vi "syrup-temp-tuner.vi"() -> ()   [LabVIEW 2013]
uses:
  <vilib>/Analysis/polynomials.llb/Scalar Polynomial Evaluation (DBL).vi
  <vilib>/Analysis/NI_AALPro.lvlib
panel:
  in  "Parameter Request":bool
  in  "Maximum Error (degF)":dbl=32.0 min=0.0 max=56.0 step=0.1
  in  "Temp Sim (degF)":dbl=32.0 min=32.0 max=1832.0 step=0.1 format="%.1f"
  in  "Hysteresis (degF)":dbl=32.0 min=0.0 max=56.0 step=0.1 format="%#.1f"
  in  "Valve Time Gain":u16=100
  in  "Min Valve On Time (ms)":u16=100
  in  "Open Valve":u8
  in  "Close Valve":u8
  in  "Auto Mode":bool
  in  "Valve On Time (ms)":u16=100
  in  "Write Tuning":bool
  in  "Temp Setpoint (degF)":dbl=32.0 min=32.0 max=1832.0 step=1.0
  out "Array":dbl[](array[numeric]) format="%.1f"
  in  "Write Setpoint":bool
  out "Waveform Chart":T1(graph)={"[0]"=63.3344, "[1]"=32.0, "[2]"=32.0, "[3]"=32.0, "[4]"=0.0, "[5]"=0.0, "[6]"=0.0, "[7]"=0.0, "[8]"=0.0}
  in  "stop":bool
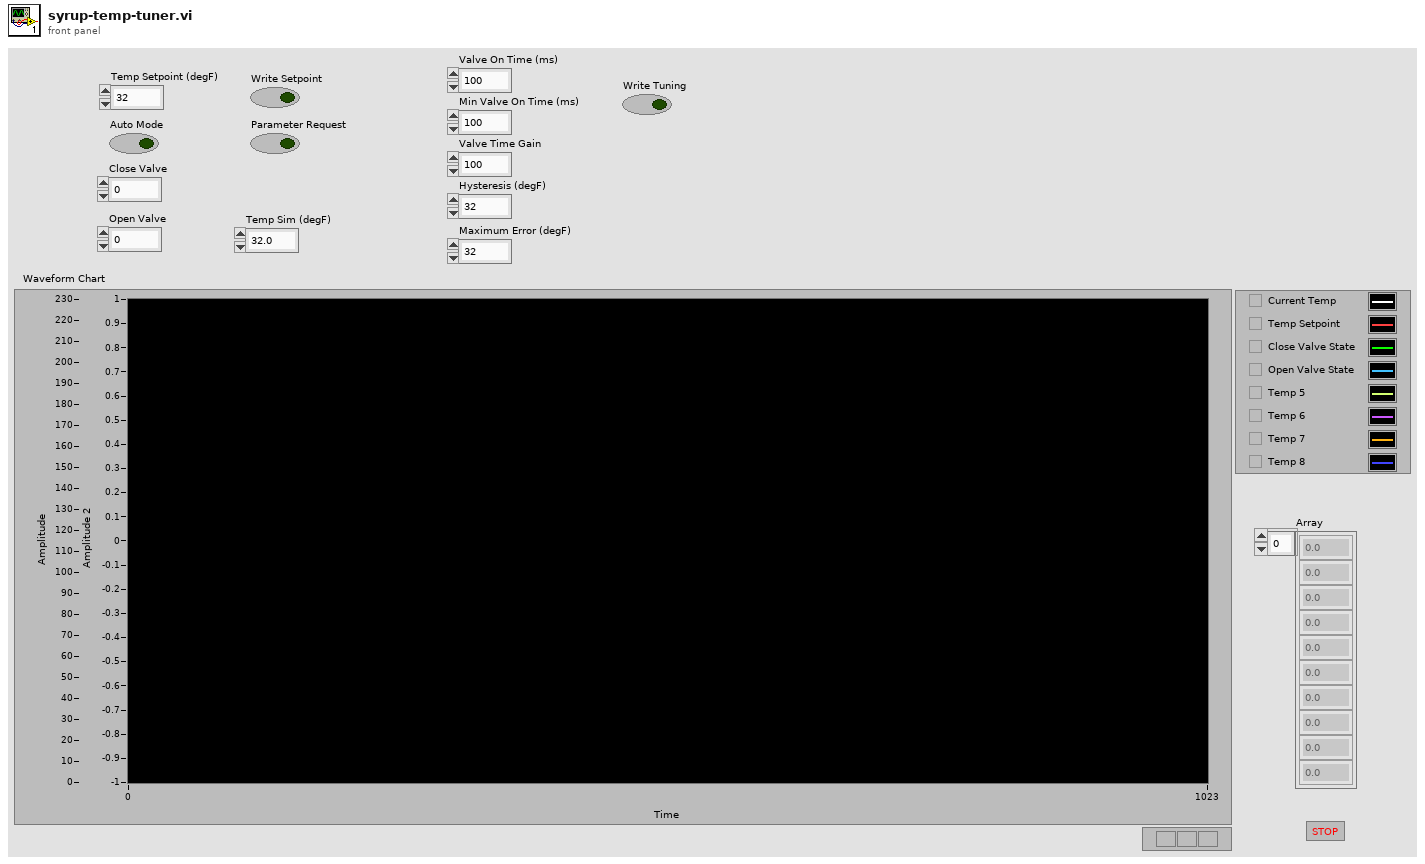
[diagram p1: front panel]
types:
  T1 = cluster{"[0]":dbl, "[1]":dbl, "[2]":dbl, "[3]":dbl, "[4]":dbl, "[5]":dbl, "[6]":dbl, "[7]":dbl, "[8]":dbl}
  T2 = enum16{"HSCAN", "MSCAN", "SWCAN", "LSFTCAN", "HSCAN2", "HSCAN3"}
  T3 = cluster{"DeviceType":i32, "Handle":i32, "NumberOfClients":i32, "SerialNumber":i32, "MaxAllowedClients":i32}[]
  T4 = cluster{"DeviceType":i32, "Handle":i32, "NumberOfClients":i32, "SerialNumber":i32, "MaxAllowedClients":i32}
  T5 = enum16{"DEVICE", "HSCAN", "MSCAN", "SWCAN", "LSFTCAN", "FORDSCP", "J1708", "JVPW", "ISO", "FIRE_HSCAN2", "FIRE_MSCAN1", "FIRE_HSCAN3", "FIRE_LIN2", "FIRE_LIN3", "FIRE_LIN4"}
  T6 = typedef "ctl spymessage.ctl" = cluster{"StatusBitField":u32, "StatusBitField2":u32, "TimeHardware":u32, "TimeHardware2":u32, "TimeSystem":u32, "TimeSystem2":u32, "TimeStampHardwareID":u8, "TimeStampHardwareID2":u8, "NetworkID":u8, "NodeID":u8, "Protocol":u8, "MessagePieceID":u8, "ColorID":u8, "NumberBytesHeader":u8, "NumberBytesData":u8, "DescriptionID":u16, "ArbIDOrHeader":u32, "Data [8]":u8[], "AckBytes [8]":u8[], "Value":sgl, "MiscData":u8}
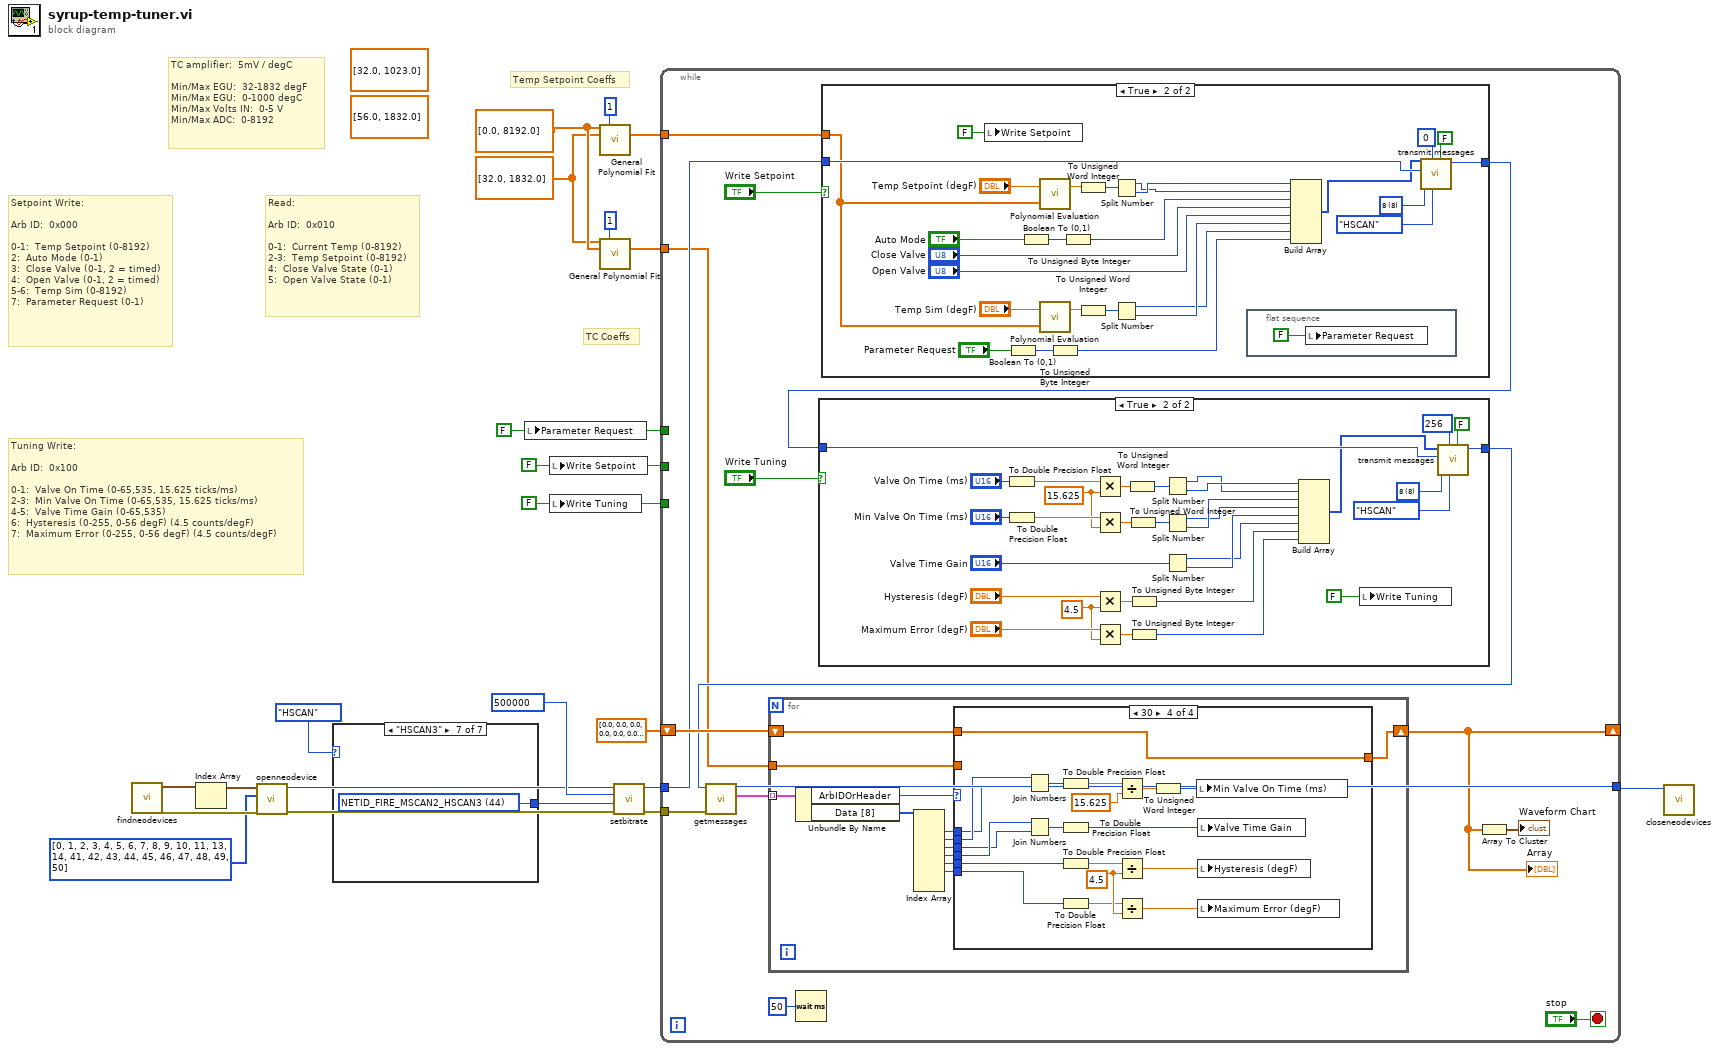
[diagram p0: block diagram]
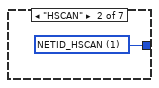
[diagram p3: hidden frame]
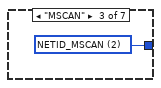
[diagram p4: hidden frame]
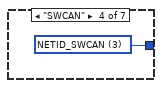
[diagram p5: hidden frame]
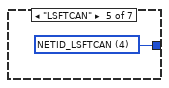
[diagram p6: hidden frame]
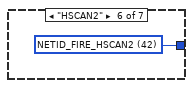
[diagram p7: hidden frame]
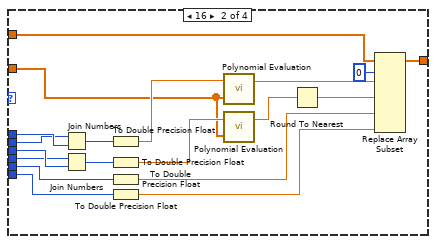
[diagram p11: hidden frame]
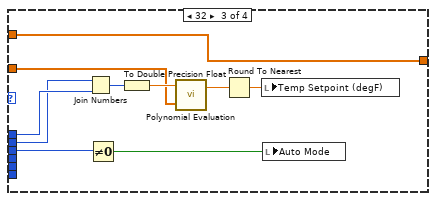
[diagram p12: hidden frame]
diagram:
  w1 = FALSE ("Send")
  (unwired) dbl[] [56.0, 1832.0] ("Y")
  (unwired) dbl[] [32.0, 1023.0] ("Y")
  w6 = FALSE ("Send")
  w2 = dbl[] [32.0, 1832.0] ("Y")
  w3 = dbl[] [0.0, 8192.0] ("Y")
  w9 = FALSE ("Send")
  w16 = 500000 items=["20000"=20000, "33333"=33333, "50000"=50000, "62500"=62500, "83333"=83333, "100000"=100000, "125000"=125000, "250000"=250000, "500000"=500000, "800000"=800000, "1000000"=1000000] ("Bit Rate")
  w19 = i8[] [0, 1, 2, 3, 4, 5, 6, 7, 8, 9, 10, 11, 13, 14, 41, 42, 43, 44, 45, 46, 47, 48, 49, 50] items=["NETID_DEVICE"=0, "NETID_HSCAN"=1, "NETID_MSCAN"=2, "NETID_SWCAN"=3, "NETID_LSFTCAN"=4, "NETID_FORDSCP"=5, "NETID_J1708"=6, "NETID_AUX"=7, "NETID_JVPW"=8, "NETID_ISO_LIN"=9, "NETID_ISOPIC"=10, "NETID_MAIN51"=11, "NETID_SCI"=13, "NETID_ISO2"=14, "NETID_FIRE_HSCAN1"=41, "NETID_FIRE_HSCAN2"=42, "NETID_FIRE_MSCAN1"=43, "NETID_FIRE_MSCAN2_HSCAN3"=44, "NETID_FIRE_SWCAN"=45, "NETID_FIRE_LSFT"=46, "NETID_FIRE_LIN1"=47, "NETID_FIRE_LIN2"=48, "NETID_FIRE_LIN3"=49, "NETID_FIRE_LIN4"=50] ("bNetworkIDs")
  # "Temp Setpoint Coeffs"
  # "TC Coeffs"
  # "TC amplifier:  5mV / degC\n\nMin/Max EGU:  32-1832 degF\nMin/Max EGU:  0-1000 degC\nMin/Max Volts IN:  0-5 V\nMin/Max ADC:  0-8192"
  # "Read:\n\nArb ID:  0x010\n\n0-1:  Current Temp (0-8192)\n2-3:  Temp Setpoint (0-8192)\n4:  Close Valve State (0-1)\n5:  Open Valve State (0-1)"
  # "Tuning Write:\n\nArb ID:  0x100\n\n0-1:  Valve On Time (0-65,535, 15.625 ticks/ms)\n2-3:  Min Valve On Time (0-65,535, 15.625 ticks/ms)\n4-5:  Valve Time Gain (0-65,535)\n6:  Hysteresis (0-255, 0-56 degF) (4.5 counts/degF)\n7:  Maximum Error (0-255, 0-56 degF) (4.5 counts/degF)"
  # "Setpoint Write:\n\nArb ID:  0x000\n\n0-1:  Temp Setpoint (0-8192)\n2:  Auto Mode (0-1)\n3:  Close Valve (0-1, 2 = timed)\n4:  Open Valve (0-1, 2 = timed)\n5-6:  Temp Sim (0-8192)\n7:  Parameter Request (0-1)"
  n1 = call "findneodevices.vi"() -> ("error out"=w21:errorcluster, "NeoDevices {}"=w22:T3)  [unwired: 3 in, 7 out]
  n2 = Index Array(array=w22) -> (element=w20:T4)  [unwired: 1 in]
  n3 = call "openneodevice.vi"("error in (no error)"=w21, "bNetworkIDs"=w19, "NeoDevice{}"=w20) -> ("error out"=w13:errorcluster, "hObject"=w14:i32)  [unwired: 2 in, 5 out]
  n4 = case shown="\"HSCAN3\"" T2."HSCAN" ("CAN Channel") {
    tunnel: [_ w23 w24 w25 w26 w27 w28] -> w15
    frame Default {
    }
    frame "HSCAN" {
      w23 = i8 1 items=["NETID_DEVICE"=0, "NETID_HSCAN"=1, "NETID_MSCAN"=2, "NETID_SWCAN"=3, "NETID_LSFTCAN"=4, "NETID_FORDSCP"=5, "NETID_J1708"=6, "NETID_AUX"=7, "NETID_JVPW"=8, "NETID_ISO_LIN"=9, "NETID_ISOPIC"=10, "NETID_MAIN51"=11, "NETID_SCI"=13, "NETID_ISO2"=14, "NETID_FIRE_HSCAN1"=41, "NETID_FIRE_HSCAN2"=42, "NETID_FIRE_MSCAN1"=43, "NETID_FIRE_MSCAN2_HSCAN3"=44, "NETID_FIRE_SWCAN"=45, "NETID_FIRE_LSFT"=46, "NETID_FIRE_LIN1"=47, "NETID_FIRE_LIN2"=48, "NETID_FIRE_LIN3"=49, "NETID_FIRE_LIN4"=50] ("NetworkID")
    }
    frame "MSCAN" {
      w24 = i8 2 items=["NETID_DEVICE"=0, "NETID_HSCAN"=1, "NETID_MSCAN"=2, "NETID_SWCAN"=3, "NETID_LSFTCAN"=4, "NETID_FORDSCP"=5, "NETID_J1708"=6, "NETID_AUX"=7, "NETID_JVPW"=8, "NETID_ISO_LIN"=9, "NETID_ISOPIC"=10, "NETID_MAIN51"=11, "NETID_SCI"=13, "NETID_ISO2"=14, "NETID_FIRE_HSCAN1"=41, "NETID_FIRE_HSCAN2"=42, "NETID_FIRE_MSCAN1"=43, "NETID_FIRE_MSCAN2_HSCAN3"=44, "NETID_FIRE_SWCAN"=45, "NETID_FIRE_LSFT"=46, "NETID_FIRE_LIN1"=47, "NETID_FIRE_LIN2"=48, "NETID_FIRE_LIN3"=49, "NETID_FIRE_LIN4"=50] ("NetworkID")
    }
    frame "SWCAN" {
      w25 = i8 3 items=["NETID_DEVICE"=0, "NETID_HSCAN"=1, "NETID_MSCAN"=2, "NETID_SWCAN"=3, "NETID_LSFTCAN"=4, "NETID_FORDSCP"=5, "NETID_J1708"=6, "NETID_AUX"=7, "NETID_JVPW"=8, "NETID_ISO_LIN"=9, "NETID_ISOPIC"=10, "NETID_MAIN51"=11, "NETID_SCI"=13, "NETID_ISO2"=14, "NETID_FIRE_HSCAN1"=41, "NETID_FIRE_HSCAN2"=42, "NETID_FIRE_MSCAN1"=43, "NETID_FIRE_MSCAN2_HSCAN3"=44, "NETID_FIRE_SWCAN"=45, "NETID_FIRE_LSFT"=46, "NETID_FIRE_LIN1"=47, "NETID_FIRE_LIN2"=48, "NETID_FIRE_LIN3"=49, "NETID_FIRE_LIN4"=50] ("NetworkID")
    }
    frame "LSFTCAN" {
      w26 = i8 4 items=["NETID_DEVICE"=0, "NETID_HSCAN"=1, "NETID_MSCAN"=2, "NETID_SWCAN"=3, "NETID_LSFTCAN"=4, "NETID_FORDSCP"=5, "NETID_J1708"=6, "NETID_AUX"=7, "NETID_JVPW"=8, "NETID_ISO_LIN"=9, "NETID_ISOPIC"=10, "NETID_MAIN51"=11, "NETID_SCI"=13, "NETID_ISO2"=14, "NETID_FIRE_HSCAN1"=41, "NETID_FIRE_HSCAN2"=42, "NETID_FIRE_MSCAN1"=43, "NETID_FIRE_MSCAN2_HSCAN3"=44, "NETID_FIRE_SWCAN"=45, "NETID_FIRE_LSFT"=46, "NETID_FIRE_LIN1"=47, "NETID_FIRE_LIN2"=48, "NETID_FIRE_LIN3"=49, "NETID_FIRE_LIN4"=50] ("NetworkID")
    }
    frame "HSCAN2" {
      w27 = i8 42 items=["NETID_DEVICE"=0, "NETID_HSCAN"=1, "NETID_MSCAN"=2, "NETID_SWCAN"=3, "NETID_LSFTCAN"=4, "NETID_FORDSCP"=5, "NETID_J1708"=6, "NETID_AUX"=7, "NETID_JVPW"=8, "NETID_ISO_LIN"=9, "NETID_ISOPIC"=10, "NETID_MAIN51"=11, "NETID_SCI"=13, "NETID_ISO2"=14, "NETID_FIRE_HSCAN1"=41, "NETID_FIRE_HSCAN2"=42, "NETID_FIRE_MSCAN1"=43, "NETID_FIRE_MSCAN2_HSCAN3"=44, "NETID_FIRE_SWCAN"=45, "NETID_FIRE_LSFT"=46, "NETID_FIRE_LIN1"=47, "NETID_FIRE_LIN2"=48, "NETID_FIRE_LIN3"=49, "NETID_FIRE_LIN4"=50] ("NetworkID")
    }
    frame "HSCAN3" {
      w28 = i8 44 items=["NETID_DEVICE"=0, "NETID_HSCAN"=1, "NETID_MSCAN"=2, "NETID_SWCAN"=3, "NETID_LSFTCAN"=4, "NETID_FORDSCP"=5, "NETID_J1708"=6, "NETID_AUX"=7, "NETID_JVPW"=8, "NETID_ISO_LIN"=9, "NETID_ISOPIC"=10, "NETID_MAIN51"=11, "NETID_SCI"=13, "NETID_ISO2"=14, "NETID_FIRE_HSCAN1"=41, "NETID_FIRE_HSCAN2"=42, "NETID_FIRE_MSCAN1"=43, "NETID_FIRE_MSCAN2_HSCAN3"=44, "NETID_FIRE_SWCAN"=45, "NETID_FIRE_LSFT"=46, "NETID_FIRE_LIN1"=47, "NETID_FIRE_LIN2"=48, "NETID_FIRE_LIN3"=49, "NETID_FIRE_LIN4"=50] ("NetworkID")
    }
  }
  n5 = local write "Parameter Request"(w1) -> ()
  n6 = local write "Write Setpoint"(w9) -> ()
  n7 = local write "Write Tuning"(w6) -> ()
  n8 = call <vilib>:"General Polynomial Fit.vi"("Y"=w3, "polynomial order"=1, "X"=w2) -> ("Polynomial Coefficients"=w4:dbl[])  [unwired: 9 in, 3 out]
  n9 = call <vilib>:"General Polynomial Fit.vi"("Y"=w2, "polynomial order"=1, "X"=w3) -> ("Polynomial Coefficients"=w5:dbl[])  [unwired: 9 in, 3 out]
  n10 = call "setbitrate.vi"("error in (no error)"=w13, "NetworkID"=w15, "BitRate"=w16, "hObject"=w14) -> ("error out"=w11:errorcluster, "hObject Out"=w12:i32)  [unwired: 6 out]
  n11 = while {
    tunnel: w12 -> [w35]
    tunnel: w11 -> [w42]
    tunnel: [w39] -> w18
    shift-right: [w36] -> _
    shift-left: dbl[] [0.0, 0.0, 0.0, 0.0, 0.0, 0.0, 0.0, 0.0] -> [w38]
    tunnel: w9 -> [_]
    tunnel: w6 -> [_]
    tunnel: w5 -> [w30]
    tunnel: w4 -> [w29]
    tunnel: w1 -> [_]
    stop <- "stop" stop-if-true
    n12 = Wait (ms)(milliseconds to wait=u32 50) -> ()  [unwired: 1 out]
    n13 = case shown="True" "Write Setpoint" {
      tunnel: w35 -> [w76 w99]
      tunnel: [w76 w97] -> w32
      tunnel: w29 -> [_ w80]
      frame False {
      }
      frame True {
        w101 = 8 items=["0", "1", "2", "3", "4", "5", "6", "7", "8", "9", "10", "11"] ("Number of \nData Bytes")
        n14 = local write "Write Setpoint"(FALSE ("Send")) -> ()
        n15 = Boolean To (0,1)(Boolean="Parameter Request") -> (0, 1=w79:i16)
        n16 = Boolean To (0,1)(Boolean="Auto Mode") -> (0, 1=w89:i16)
        n17 = call-poly <vilib>:"Polynomial Evaluation.vi"("P(x)"=w80, "a"="Temp Setpoint (degF)") -> ("P(a)"=w95:dbl)  [unwired: 1 out]
        n18 = call-poly <vilib>:"Polynomial Evaluation.vi"("P(x)"=w80, "a"="Temp Sim (degF)") -> ("P(a)"=w84:dbl)  [unwired: 1 out]
        n19 = To Unsigned Byte Integer(number=w79) -> (unsigned 8bit integer=w77:u8)
        n20 = To Unsigned Byte Integer(number=w89) -> (unsigned 8bit integer=w88:u8)
        n21 = To Unsigned Word Integer(number=w95) -> (unsigned 16bit integer=w93:u16)
        n22 = To Unsigned Word Integer(number=w84) -> (unsigned 16bit integer=w85:u16)
        n23 = Split Number(x=w93) -> (hi(x)=w91:u8, lo(x)=w92:u8)
        n24 = Split Number(x=w85) -> (hi(x)=w81:u8, lo(x)=w82:u8)
        n25 = flat-sequence {
          frame #0 {
            n26 = local write "Parameter Request"(FALSE ("Send")) -> ()
          }
        }
        n27 = Build Array(w92, w91, w88, "Close Valve", "Open Valve", w82, w81, w77) -> (w94:u8[])
        n28 = call "transmit messages.vi"("extended ID?"=FALSE ("Send Extended ID"), "Network"=T5."HSCAN", "Arb ID"=u32 0, "Number of \nData Bytes"=w101, "hObject In"=w99, "Data"=w94) -> ("hObject Out"=w97:i32)  [unwired: 1 in, 4 out]
      }
    }
    n29 = case shown="True" "Write Tuning" {
      tunnel: w32 -> [w44 w71]
      tunnel: [w44 w69] -> w31
      frame False {
      }
      frame True {
        w47 = 4.5 ("y")
        w48 = 15.625 ("y")
        w73 = 8 items=["0", "1", "2", "3", "4", "5", "6", "7", "8", "9", "10", "11"] ("Number of \nData Bytes")
        n30 = To Double Precision Float(number="Valve On Time (ms)") -> (double precision float=w64:dbl)
        n31 = To Double Precision Float(number="Min Valve On Time (ms)") -> (double precision float=w63:dbl)
        n32 = Multiply(x=w64, y=w48) -> (x*y=w46:dbl)
        n33 = Multiply(x=w63, y=w48) -> (x*y=w62:dbl)
        n34 = Multiply(x="Hysteresis (degF)", y=w47) -> (x*y=w57:dbl)
        n35 = Multiply(x="Maximum Error (degF)", y=w47) -> (x*y=w51:dbl)
        n36 = To Unsigned Word Integer(number=w46) -> (unsigned 16bit integer=w45:u16)
        n37 = To Unsigned Word Integer(number=w62) -> (unsigned 16bit integer=w60:u16)
        n38 = To Unsigned Byte Integer(number=w57) -> (unsigned 8bit integer=w52:u8)
        n39 = To Unsigned Byte Integer(number=w51) -> (unsigned 8bit integer=w49:u8)
        n40 = Split Number(x=w45) -> (hi(x)=w67:u8, lo(x)=w68:u8)
        n41 = Split Number(x=w60) -> (hi(x)=w55:u8, lo(x)=w56:u8)
        n42 = Split Number(x="Valve Time Gain") -> (hi(x)=w53:u8, lo(x)=w54:u8)
        n43 = Build Array(w68, w67, w56, w55, w54, w53, w52, w49) -> (w66:u8[])
        n44 = local write "Write Tuning"(FALSE ("Send")) -> ()
        n45 = call "transmit messages.vi"("extended ID?"=FALSE ("Send Extended ID"), "Network"=T5."HSCAN", "Arb ID"=u32 256, "Number of \nData Bytes"=w73, "hObject In"=w71, "Data"=w66) -> ("hObject Out"=w69:i32)  [unwired: 1 in, 4 out]
      }
    }
    n46 = call "getmessages.vi"("error in (no error)"=w42, "hObject"=w31) -> ("pMsgs"=w43:T6[], "hObject Out"=w39:i32)  [unwired: 8 out]
    n47 = for {
      tunnel: w43 -> [w116] mode=indexing
      shift-right: [w111] -> w36
      shift-left: w38 -> [w112]
      tunnel: w30 -> [w107]
      n48 = Unbundle By Name(w116) -> ("ArbIDOrHeader"=w105:u32, "Data [8]"=w115:u8[])
      n49 = Index Array(array=w115) -> (element #1=w114:u8, element #2=w113:u8, element #3=w110:u8, element #4=w109:u8, element #5=w108:u8, element #6=w106:u8)  [unwired: 8 in, 2 out]
      n50 = case shown="30" w105 {
        tunnel: w114 -> [_ w136 w139 w161]
        tunnel: w113 -> [_ w135 w138 w162]
        tunnel: w112 -> [w117 w134 w146 w164]
        tunnel: [w117 w132 w146 w164] -> w111
        tunnel: w110 -> [_ w129 w137 w155]
        tunnel: w109 -> [_ w128 _ w156]
        tunnel: w108 -> [_ w127 _ w154]
        tunnel: w107 -> [_ w125 w140 _]
        tunnel: w106 -> [_ w123 _ w150]
        frame Default {
        }
        frame 16 {
          n51 = Join Numbers(hi=w135, lo=w136) -> ((hi.lo)=w131:u16)
          n52 = Join Numbers(hi=w128, lo=w129) -> ((hi.lo)=w130:u16)
          n53 = To Double Precision Float(number=w131) -> (double precision float=w133:dbl)
          n54 = To Double Precision Float(number=w130) -> (double precision float=w126:dbl)
          n55 = To Double Precision Float(number=w127) -> (double precision float=w124:dbl)
          n56 = To Double Precision Float(number=w123) -> (double precision float=w122:dbl)
          n57 = call-poly <vilib>:"Polynomial Evaluation.vi"("P(x)"=w125, "a"=w133) -> ("P(a)"=w120:dbl)  [unwired: 1 out]
          n58 = call-poly <vilib>:"Polynomial Evaluation.vi"("P(x)"=w125, "a"=w126) -> ("P(a)"=w119:dbl)  [unwired: 1 out]
          n59 = Round To Nearest(number=w119) -> (nearest integer value=w118:dbl)
          n60 = Replace Array Subset(array=w134, new element #1=w120, index #1=0 ("index"), new element #2=w118, new element #3=w124, new element #4=w122) -> (w132:dbl[])  [unwired: 3 in]
        }
        frame 32 {
          n61 = Join Numbers(hi=w138, lo=w139) -> ((hi.lo)=w141:u16)
          n62 = Not Equal To 0?(x=w137) -> (x != 0?=w143:bool)
          n63 = To Double Precision Float(number=w141) -> (double precision float=w142:dbl)
          n64 = call-poly <vilib>:"Polynomial Evaluation.vi"("P(x)"=w140, "a"=w142) -> ("P(a)"=w144:dbl)  [unwired: 1 out]
          n65 = Round To Nearest(number=w144) -> (nearest integer value=w145:dbl)
          n66 = local write "Temp Setpoint (degF)"(w145) -> ()
          n67 = local write "Auto Mode"(w143) -> ()
        }
        frame 48 {
          w151 = 4.5 ("y")
          n68 = Join Numbers(hi=w162, lo=w161) -> ((hi.lo)=w163:u16)
          n69 = Join Numbers(hi=w156, lo=w155) -> ((hi.lo)=w147:u16)
          n70 = To Double Precision Float(number=w163) -> (double precision float=w160:dbl)
          n71 = To Double Precision Float(number=w147) -> ()  [unwired: 1 out]
          n72 = To Double Precision Float(number=w154) -> (double precision float=w153:dbl)
          n73 = To Double Precision Float(number=w150) -> (double precision float=w149:dbl)
          n74 = Divide(x=w160, y=15.625) -> (x/y=w159:dbl)
          n75 = Divide(x=w153, y=w151) -> (x/y=w152:dbl)
          n76 = Divide(x=w149, y=w151) -> (x/y=w148:dbl)
          n77 = To Unsigned Word Integer(number=w159) -> (unsigned 16bit integer=w158:u16)
          n78 = local write "Min Valve On Time (ms)"(w158) -> ()
          n79 = local write "Valve Time Gain"(w147) -> ()
          n80 = local write "Hysteresis (degF)"(w152) -> ()
          n81 = local write "Maximum Error (degF)"(w148) -> ()
        }
      }
    }
    "Array" <- w36
    n82 = Array To Cluster(array=w36) -> (cluster=→"Waveform Chart":T1)
  }
  n83 = call "closeneodevices.vi"("hObject"=w18) -> ()  [unwired: 2 in, 9 out]
